vi "Motor_Write_Refnum.vi"(8 "Motor_Dev_Ref":T1, 9 "Shooter_Motor_1":dbl, 10 "Intake_Stage":dbl, 11 "Intake_1":dbl) -> ()   [LabVIEW 2015]
uses:
  Ref_Num/Motor_Type_Def.ctl
  <vilib>/Rock Robotics/WPI/RobotDrive/WPI_RobotDriveDevRef.ctl
  <vilib>/Rock Robotics/WPI/MotorControl/WPI_MotorControlDeviceRef.ctl
  <vilib>/Rock Robotics/WPI/MotorControl/WPI_MotorControlType.ctl
  <vilib>/Rock Robotics/SystemInterfaces/DIO/FPGA_DIOPWMChannel.ctl
  <vilib>/Rock Robotics/WPI/PWM/WPI_PWMDeadband.ctl
  <vilib>/Rock Robotics/WPI/CAN/Jaguar/SubVIs/WPI_CANJaguar_ControlMode.ctl
  <vilib>/Rock Robotics/WPI/CAN/TalonSRX/WPI_CANTalonSRX_APIControlMode.ctl
panel:
  # "Created by Matt Carr on 1/30/2016"
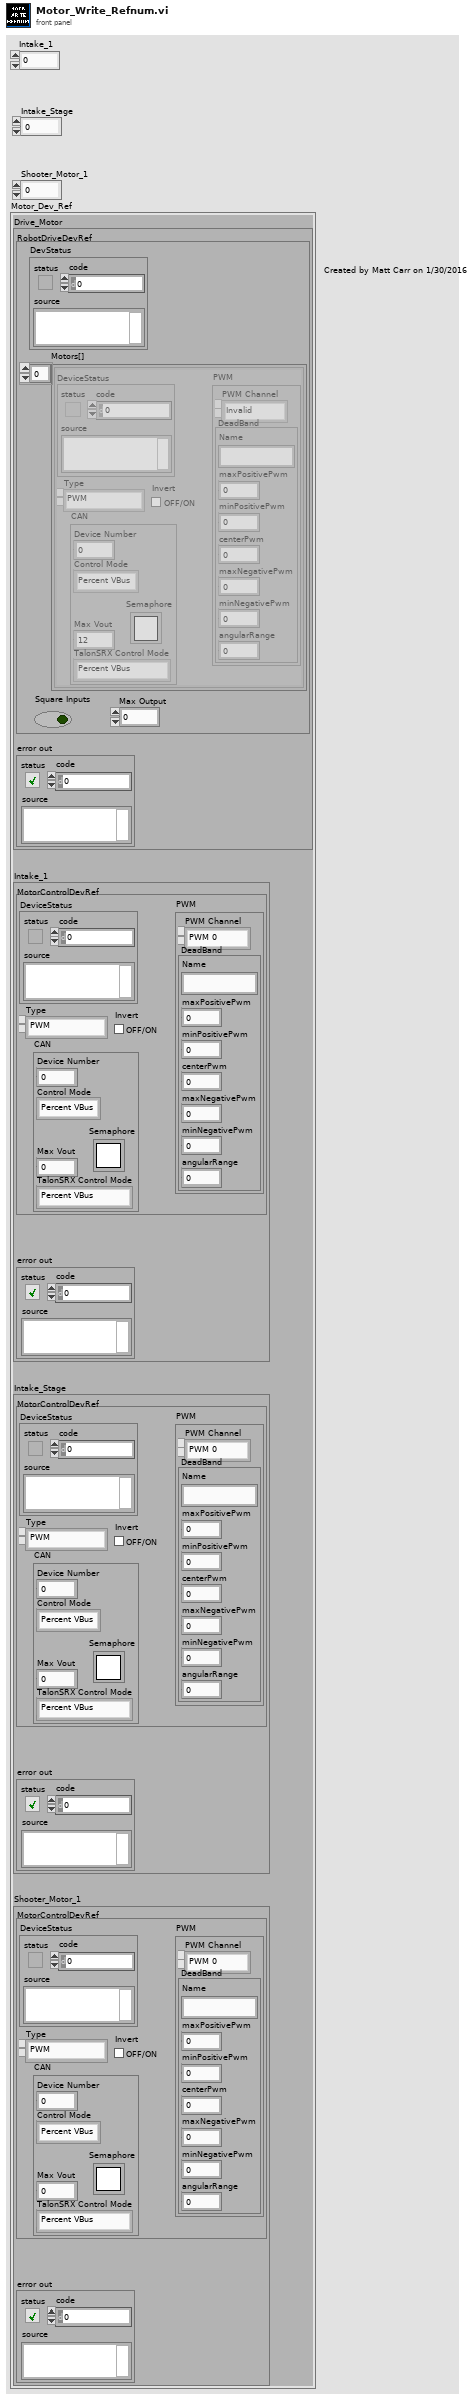
[diagram p1: front panel]
types:
  T1 = typedef "Motor_Type_Def.ctl" = cluster{"Drive_Motor":cluster{"RobotDriveDevRef":T2, "error out":errorcluster}, "Intake_1":cluster{"MotorControlDevRef":T3, "error out":errorcluster}, "Intake_Stage":cluster{"MotorControlDevRef":T3, "error out":errorcluster}, "Shooter_Motor_1":cluster{"MotorControlDevRef":T3, "error out":errorcluster}}
  T2 = typedef "WPI_RobotDriveDevRef.ctl" = cluster{"DevStatus":errorcluster, "Motors[]":T3[], "Square Inputs":bool, "Max Output":dbl}
  T3 = typedef "WPI_MotorControlDeviceRef.ctl" = cluster{"DeviceStatus":errorcluster, "Type":T4, "PWM":cluster{"PWM Channel":T5, "DeadBand":T6}, "CAN":cluster{"Device Number":u8, "Control Mode":T7, "Semaphore":T8, "Max Vout":dbl, "TalonSRX Control Mode":T9}, "Invert":bool}
  T4 = typedef "WPI_MotorControlType.ctl" = enum16{"PWM", "CAN", "CANTalonSRX"}
  T5 = typedef "FPGA_DIOPWMChannel.ctl" = enum8{"PWM 0", "PWM 1", "PWM 2", "PWM 3", "PWM 4", "PWM 5", "PWM 6", "PWM 7", "PWM 8", "PWM 9", "PWM MXP 0", "PWM MXP 1", "PWM MXP 2", "PWM MXP 3", "PWM MXP 4", "PWM MXP 5", "PWM MXP 6", "PWM MXP 7", "PWM MXP 8", "PWM MXP 9", "Invalid"}
  T6 = typedef "WPI_PWMDeadband.ctl" = cluster{"Name":string, "maxPositivePwm":i32, "minPositivePwm":i32, "centerPwm":i32, "maxNegativePwm":i32, "minNegativePwm":i32, "angularRange":u16}
  T7 = typedef "WPI_CANJaguar_ControlMode.ctl" = enum8{"Percent VBus", "Current", "Speed", "Position", "Voltage"}
  T8 = typedef "Semaphore RefNum" = refnum<k1>
  T9 = typedef "WPI_CANTalonSRX_APIControlMode.ctl" = enum8{"Percent VBus", "Speed", "Position", "Slave", "Unchanged / Invalid", "Voltage Compensation", "Current", "Motion Profile"}
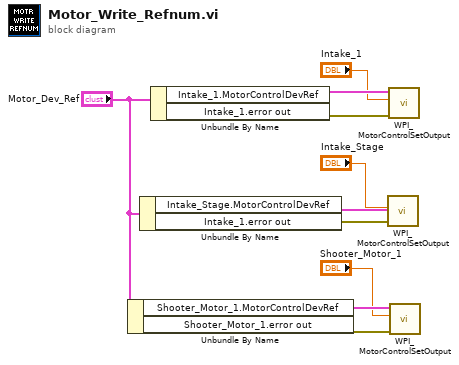
[diagram p0: block diagram]
diagram:
  n1 = Unbundle By Name("Motor_Dev_Ref") -> ("Shooter_Motor_1.MotorControlDevRef"=w4:T3, "Shooter_Motor_1.error out"=w3:errorcluster)
  n2 = Unbundle By Name("Motor_Dev_Ref") -> ("Intake_Stage.MotorControlDevRef"=w7:T3, "Intake_1.error out"=w6:errorcluster)
  n3 = Unbundle By Name("Motor_Dev_Ref") -> ("Intake_1.MotorControlDevRef"=w10:T3, "Intake_1.error out"=w9:errorcluster)
  n4 = call <vilib>:"WPI_MotorControlSetOutput.vi"("error in (no error)"=w6, "Output"="Intake_Stage", "MotorControlDevRef"=w7) -> ()  [unwired: 6 in, 3 out]
  n5 = call <vilib>:"WPI_MotorControlSetOutput.vi"("error in (no error)"=w9, "Output"="Intake_1", "MotorControlDevRef"=w10) -> ()  [unwired: 6 in, 3 out]
  n6 = call <vilib>:"WPI_MotorControlSetOutput.vi"("error in (no error)"=w3, "Output"="Shooter_Motor_1", "MotorControlDevRef"=w4) -> ()  [unwired: 6 in, 3 out]
